vi "Sagar_ToFile(glue).vi"(0 "Module ID":string="Test", 7 "Assembler Names":string="Sagar", 8 "Module reports file path":path, 9 "Glue Batch ID":string="Test", 10 "Write to file":bool=TRUE, 11 "error in (no error)":errorcluster) -> (19 "error out":errorcluster)   [LabVIEW 2016]
uses:
  <vilib>/Utility/config.llb/Write Key (String).vi
  <vilib>/Utility/config.llb/NI_LVConfig.lvlib
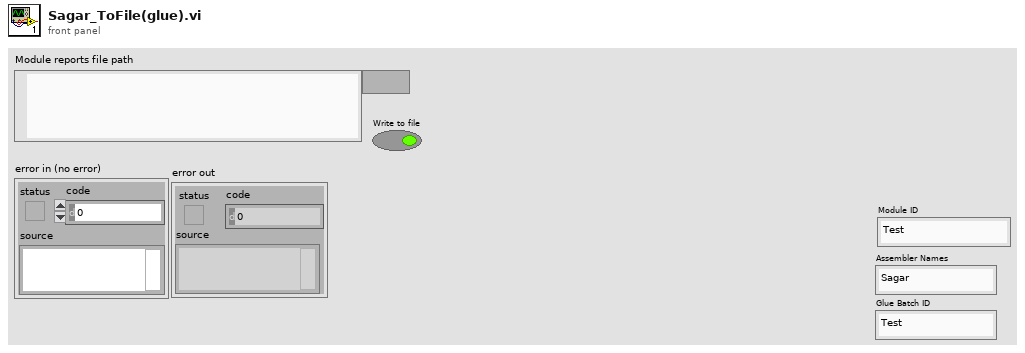
[diagram p1: front panel]
types:
  T1 = typedef "NI_LVConfig.lvlib/Config Data RefNum.ctl" = refnum<k1>
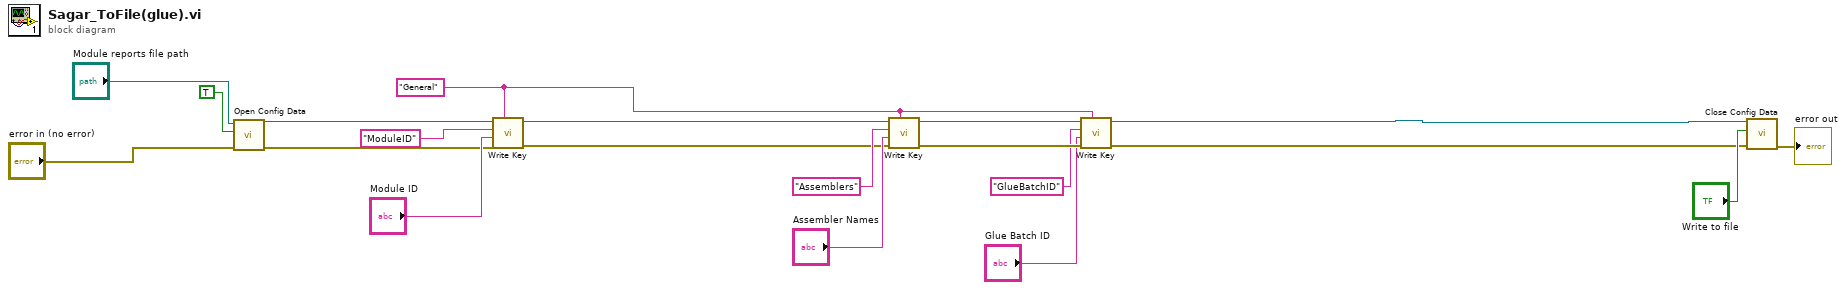
[diagram p0: block diagram]
diagram:
  w11 = "General" ("section")
  n1 = call <vilib>:"Open Config Data.vi"("error in (no error)"="error in (no error)", "create file if necessary (T)"=TRUE, "configuration file path"="Module reports file path") -> ("error out"=w14:errorcluster, "refnum"=w17:T1)  [unwired: 6 in, 1 out]
  n2 = call-poly <vilib>:"Write Key.vi"("section"=w11, "error in (no error)"=w14, "value"="Module ID", "key"="ModuleID", "refnum"=w17) -> ("error out"=w2:errorcluster, "refnum out"=w3:T1)  [unwired: 4 in, 1 out]
  n3 = call-poly <vilib>:"Write Key.vi"("section"=w11, "error in (no error)"=w2, "value"="Assembler Names", "key"="Assemblers", "refnum"=w3) -> ("error out"=w9:errorcluster, "refnum out"=w10:T1)  [unwired: 4 in, 1 out]
  n4 = call-poly <vilib>:"Write Key.vi"("section"=w11, "error in (no error)"=w9, "value"="Glue Batch ID", "key"="GlueBatchID", "refnum"=w10) -> ("error out"=w1:errorcluster, "refnum out"=w4:T1)  [unwired: 4 in, 1 out]
  n5 = call <vilib>:"Close Config Data.vi"("error in (no error)"=w1, "write file if changed (T)"="Write to file", "refnum"=w4) -> ("error out"=→"error out":errorcluster)  [unwired: 7 in, 1 out]
